vi "Choose Retical.vi"(10 "Image In":T2, 11 "Climb Retical":bool) -> (3 "Image Out":T2)   [LabVIEW 2012]
uses:
  <vilib>/vision/Image Controls.llb/IMAQ Image.ctl
panel:
  in  "Color":u32(colorbox)=16711680
  in  "Rectangle":T1={"Left"=125, "Top"=70, "Right"=195, "Bottom"=90}
  in  "Climb Begin":cluster{"X":i32, "Y":i32}
  in  "Climb End":cluster{"X":i32, "Y":i32}
  in  "Start Point":cluster{"X":i32, "Y":i32}
  in  "End Point":cluster{"X":i32, "Y":i32}
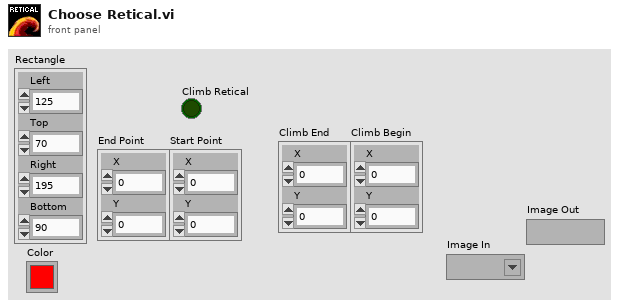
[diagram p1: front panel]
types:
  T1 = cluster{"Left":i32, "Top":i32, "Right":i32, "Bottom":i32}
  T2 = typedef "IMAQ Image.ctl" = refnum<image>
  T3 = enum16{"Shooting Rect", "Pin Shooting", "Climbing"}
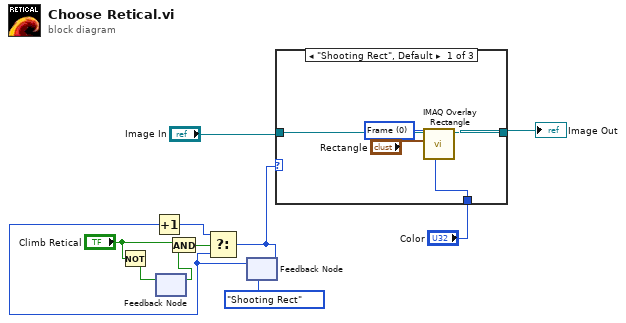
[diagram p0: block diagram]
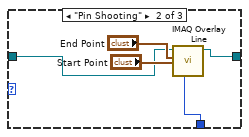
[diagram p2: hidden frame]
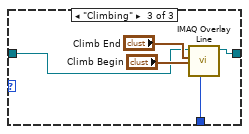
[diagram p3: hidden frame]
diagram:
  n1 = Not(x="Climb Retical") -> (.not. x?=w7:bool)
  n2 = feedback #1() -> (w8:bool)  [unwired: 1 in]
  n3 = feedback-in #1(w7) -> ()
  n4 = And(x="Climb Retical", y=w8) -> (x .and. y?=w6:bool)
  n5 = feedback #2(T3."Shooting Rect" ("Enum")) -> (w3:T3)
  n6 = Increment(x=w3) -> (x+1=w5:T3)
  n7 = Select(t=w5, s=w6, f=w3) -> (s? t:f=w1:T3)
  n8 = feedback-in #2(w1) -> ()
  n9 = case shown="\"Shooting Rect\", Default" w1 {
    tunnel: "Image In" -> [w15 w19 w24]
    tunnel: [w14 w18 w23] -> w10
    tunnel: "Color" -> [w13 w17 w22]
    frame "Shooting Rect", Default {
      w12 = u32 0 items=["Frame", "Fill", "Highlight"] ("Drawing Mode (Frame)")
      n10 = call "IMAQ Overlay Rectangle"("Color"=w13, "Drawing Mode (Frame)"=w12, "Rectangle"="Rectangle", "Image"=w15) -> ("Image Out"=w14:T2)  [unwired: 6 in, 1 out]
    }
    frame "Pin Shooting" {
      n11 = call "IMAQ Overlay Line"("Color"=w17, "End Point"="Start Point", "Start Point"="End Point", "Image"=w19) -> ("Image Out"=w18:T2)  [unwired: 6 in, 1 out]
    }
    frame "Climbing" {
      n12 = call "IMAQ Overlay Line"("Color"=w22, "End Point"="Climb Begin", "Start Point"="Climb End", "Image"=w24) -> ("Image Out"=w23:T2)  [unwired: 6 in, 1 out]
    }
  }
  "Image Out" <- w10
